vi "Sword_Create.vi"(8 "Error In":errorcluster, 10 "Enchantment":refnum<class "IEnchantment.lvclass">, 11 "reference in":refnum<class "Sword.lvclass">) -> (0 "Error Out":errorcluster, 3 "reference out":refnum<class "Sword.lvclass">)   [LabVIEW 2020, in "Sword.lvclass"]
uses:
  Sword.lvclass
  Sword.lvclass/Sword.ctl
  IEnchantment_interface/IEnchantment.lvclass
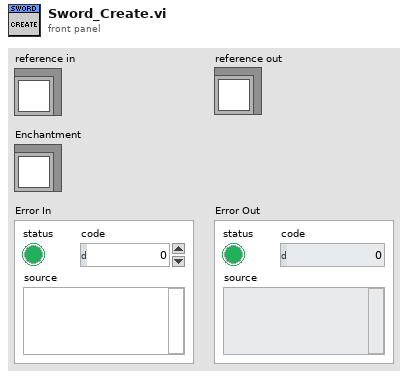
[diagram p1: front panel]
types:
  T1 = typedef "Sword.lvclass/ObjectAttributes.ctl" = cluster{"_enchantment":refnum<class "IEnchantment.lvclass">}
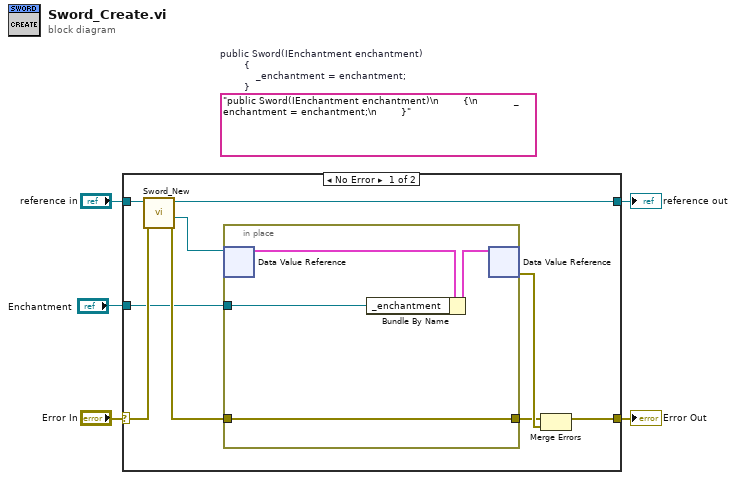
[diagram p0: block diagram]
diagram:
  (unwired) "public Sword(IEnchantment enchantment)\n        {\n            _enchantment = enchantment;\n        }"  # public Sword(IEnchantment enchantment)         {             _enchantment = enchantment;         }
  n1 = case shown="No Error" "Error In" {
    selector: "Error In" -> [w13 w20]
    tunnel: [w7 w20] -> w4
    tunnel: "reference in" -> [w14 w19]
    tunnel: [w12 w19] -> w2
    tunnel: "Enchantment" -> [w6 _]
    frame No Error {
      n2 = call "Sword_New.vi"("error in (no error)"=w13, "reference in"=w14) -> ("error out"=w9:errorcluster, "DVRRefOut"=w10:refnum<data-value>, "reference out"=w12:refnum<class "Sword.lvclass">)  [unwired: 6 in, 1 out]
      n3 = in-place {
        in-place-border: w9 -> [w16]
        in-place-border: [w16] -> w8
        in-place-border: w6 -> [w15]
        n4 = in-place-dvr #1(w10) -> (w17:T1)  [unwired: 1 out]
        n5 = Bundle By Name(cluster=w17, "_enchantment"=w15) -> (w18:T1)
        n6 = in-place-dvr #1(w18) -> (w11:errorcluster)  [unwired: 1 out]
      }
      n7 = Merge Errors(w8, w11) -> (w7:errorcluster)
    }
    frame Error {
      # "VI-TechBaseTemplate_Simple_4x4x4"
    }
  }
  "Error Out" <- w4
  "reference out" <- w2
